vi "Create ECU.vi"(4 "Error In":errorcluster, 7 "reference in":refnum<class "Diesel Engine Factory.lvclass">) -> (0 "Error Out":errorcluster, 2 "IECU":refnum<class "IECU.lvclass">, 3 "reference out":refnum<class "Diesel Engine Factory.lvclass">)   [LabVIEW 2024, in "Diesel Engine Factory.lvclass"]
uses:
  Diesel Engine Factory.lvclass
  Product Folder/IECU/IECU.lvclass
  Diesel Engine Factory.lvclass/Diesel Engine Factory.ctl
  Product Folder/Diesel ECU/Diesel ECU.lvclass
  C:/Users/burakkorkmaz/Desktop/Leveling/labview-desing-patterns/Abstract Factory Pattern/Product Folder/Diesel ECU/Diesel ECU.lvclass
  C:/Users/burakkorkmaz/Desktop/Leveling/labview-desing-patterns/Abstract Factory Pattern/Product Folder/IECU/IECU.lvclass
panel:
  # "Connector Pane"
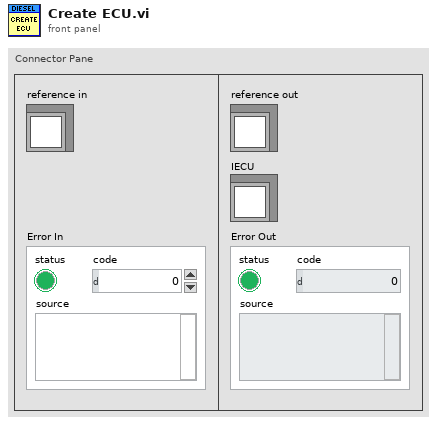
[diagram p1: front panel]
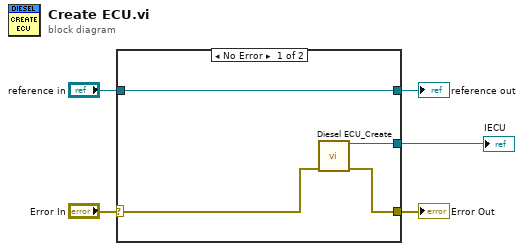
[diagram p0: block diagram]
diagram:
  n1 = case shown="No Error" "Error In" {
    selector: "Error In" -> [w9 w11]
    tunnel: [w7 w11] -> w4
    tunnel: [w8 w10] -> w2
    tunnel: "reference in" -> [w8 w10]
    tunnel: [w6 _] -> w1
    frame No Error {
      n2 = call "Diesel ECU_Create.vi"("Error In"=w9) -> ("reference out"=w6:refnum<class "Diesel ECU.lvclass">, "Error Out"=w7:errorcluster)  [unwired: 13 in]
    }
    frame Error {
    }
  }
  "Error Out" <- w4
  "reference out" <- w2
  "IECU" <- w1
